vi "CRYGet Main Menu Recent.vi"(10 "Menu TAG":string, 11 "RecentFiles":path) -> (1 "Seq Result":bool, 2 "Seq Item Tags Out":string[](array[string]), 3 "Seq Item Names Out":string[](array[string]))   [LabVIEW 2013]
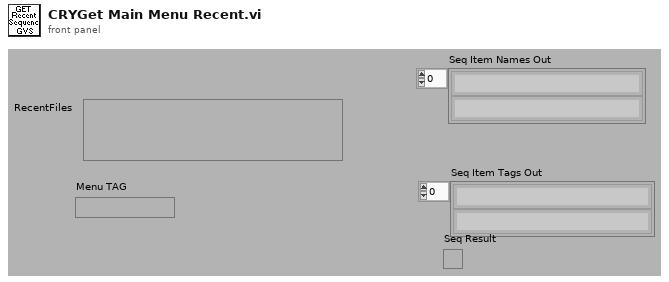
[diagram p1: front panel]
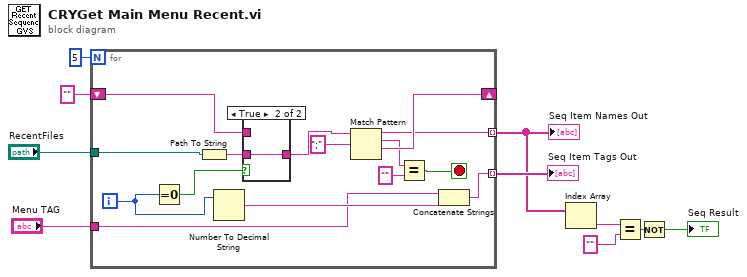
[diagram p0: block diagram]
diagram:
  n1 = for {
    N: 5 -> [_]
    shift-right: [w21] -> _
    shift-left: "" -> [w20]
    tunnel: [w17] -> w8 mode=indexing
    tunnel: [w14] -> w9 mode=indexing
    tunnel: "RecentFiles" -> [w12]
    tunnel: "Menu TAG" -> [w11]
    i -> [w15]
    stop <- w13 stop-if-true
    n2 = Equal To 0?(x=w15) -> (x = 0?=w24:bool)
    n3 = Path To String(path=w12) -> (string=w25:string)
    n4 = Number To Decimal String(number=w15) -> (decimal integer string=w16:string)  [unwired: 1 out]
    n5 = case shown="True" w24 {
      tunnel: w25 -> [_ w27]
      tunnel: [w26 w27] -> w22
      tunnel: w20 -> [w26 _]
      frame False {
      }
      frame True {
      }
    }
    n6 = Match Pattern(string=w22, regular expression=";" ("search string")) -> (before substring=w17:string, match substring=w19:string, after substring=w21:string)  [unwired: 2 out]
    n7 = Equal?(x=w19, y="") -> (x = y?=w13:bool)
    n8 = Concatenate Strings(w11, w16) -> (w14:string)
  }
  "Seq Item Names Out" <- w8
  "Seq Item Tags Out" <- w9
  n9 = Index Array(array=w8) -> (element=w7:string)  [unwired: 1 in]
  n10 = Equal?(x=w7, y="") -> (x = y?=w5:bool)
  n11 = Not(x=w5) -> (.not. x?=→"Seq Result":bool)
